vi "Set Active Chal ID.vi"(8 "error in (no error)":errorcluster, 11 "Active Chal ID":i64) -> (0 "error out":errorcluster)   [LabVIEW 2020, in "Scores.lvclass"]
uses:
  Scores.lvclass
  Scores.lvclass/Scores.ctl
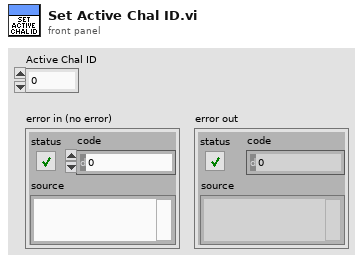
[diagram p1: front panel]
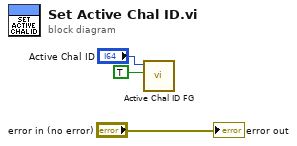
[diagram p0: block diagram]
diagram:
  n1 = call "Active Chal ID FG.vi"("Set?"=TRUE, "Active Chal ID In"="Active Chal ID") -> ()  [unwired: 9 in, 1 out]
  "error out" <- "error in (no error)"
